vi "신호시뮬레이션(열거형).vi"() -> ()   [LabVIEW 2014]
uses:
  <vilib>/Analysis/NI_AALBase.lvlib
panel:
  in  "정지":bool
  in  "열거형":T1(ring)
  out "웨이브폼 그래프":dbl[](graph)
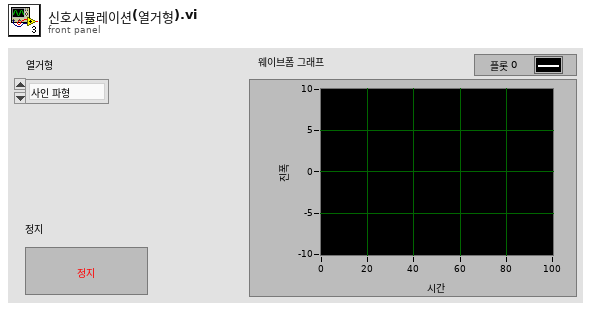
[diagram p1: front panel]
types:
  T1 = enum16{"사인 파형", "삼각 파형", "사각 파형", "톱니 파형", "노이즈"}
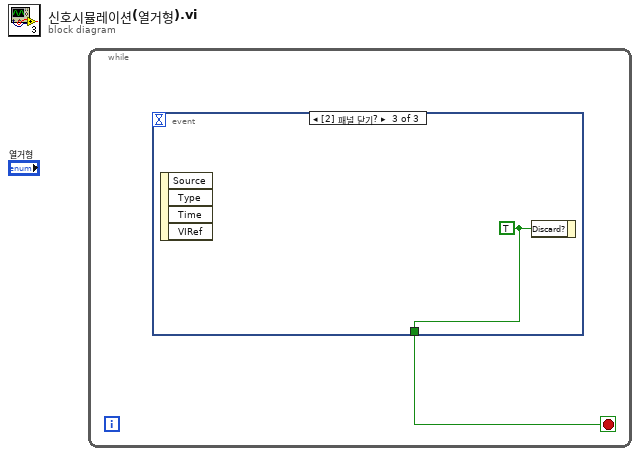
[diagram p0: block diagram]
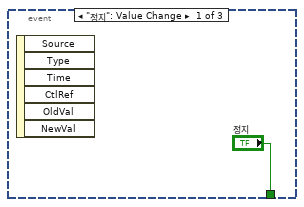
[diagram p2: hidden frame]
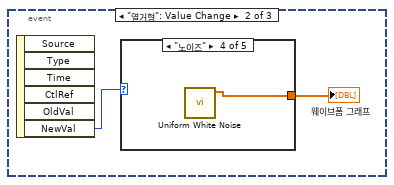
[diagram p3: hidden frame]
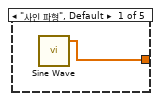
[diagram p4: hidden frame]
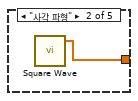
[diagram p5: hidden frame]
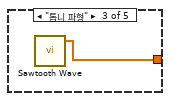
[diagram p6: hidden frame]
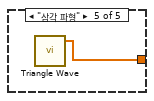
[diagram p7: hidden frame]
diagram:
  n1 = while {
    stop <- w1 stop-if-true
    n2 = event shown="[2] 패널 닫기?" {
      selector: _ -> [_ _ _]
      dyn-events: _ -> [_ _ _]
      timeout: _ -> [_ _ _]
      tunnel: ["정지" _ w10] -> w1
      event "정지": Value Change {
        n3 = event-data() -> ()  [unwired: 1 in, 6 out]
      }
      event "열거형": Value Change {
        n4 = event-data() -> ("NewVal"=w4:T1)  [unwired: 1 in, 5 out]
        n5 = case shown="\"노이즈\"" w4 {
          tunnel: [w5 w6 w7 w8 w9] -> w3
          frame "사인 파형", Default {
            n6 = call <vilib>:"Sine Wave.vi"() -> ("sine wave"=w5:dbl[])  [unwired: 5 in, 2 out]
          }
          frame "사각 파형" {
            n7 = call <vilib>:"Square Wave.vi"() -> ("square wave"=w6:dbl[])  [unwired: 6 in, 2 out]
          }
          frame "톱니 파형" {
            n8 = call <vilib>:"Sawtooth Wave.vi"() -> ("sawtooth wave"=w7:dbl[])  [unwired: 5 in, 2 out]
          }
          frame "노이즈" {
            n9 = call <vilib>:"Uniform White Noise.vi"() -> ("uniform white noise"=w8:dbl[])  [unwired: 10 in, 1 out]
          }
          frame "삼각 파형" {
            n10 = call <vilib>:"Triangle Wave.vi"() -> ("triangle wave"=w9:dbl[])  [unwired: 5 in, 2 out]
          }
        }
        "웨이브폼 그래프" <- w3
      }
      event Panel Close? {
        w10 = TRUE ("버림?")
        n11 = event-data() -> ()  [unwired: 1 in, 4 out]
        n12 = event-data("Discard?"=w10) -> ()  [unwired: 1 in, 1 out]
      }
    }
  }
